vi "Init Interface.vi"(8 "error in":errorcluster, 9 "Config Section":string, 10 "hse-config":refnum<class "config-base.lvclass">, 11 "DB-SQLite":refnum<class "DB-SQLite.lvclass">) -> (0 "error out":errorcluster, 3 "DB-SQLite":refnum<class "DB-SQLite.lvclass">)   [LabVIEW 2020, in "hse-db-sqlite.lvlib" / "DB-SQLite.lvclass"]
doc: "____\nHAMPEL SOFTWARE ENGINEERING v1.4.0 (2023-12-19 09:52)"
uses:
  DB-SQLite.lvclass
  hse-libraries/Source/hse-configuration/config-base/config-base.lvclass
  hse-libraries/Source/hse-application/hse-application.lvclass/hse-application.ctl
  hse-libraries/Source/hse-application/HSE Application not initialized--error.vi
  hse-libraries/Source/hse-application/hse-application__GetSingleton.vi
  <vilib>/Utility/sysdir.llb/Get System Directory.vi
  <vilib>/Utility/error.llb/Error Cluster From Error Code.vi
  DB-SQLite.lvclass/DB-SQLite.ctl
  hse-libraries/Source/hse-application/hse-application.lvclass
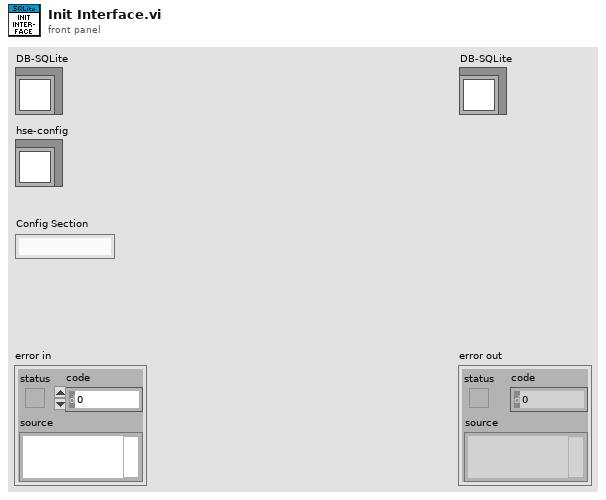
[diagram p1: front panel]
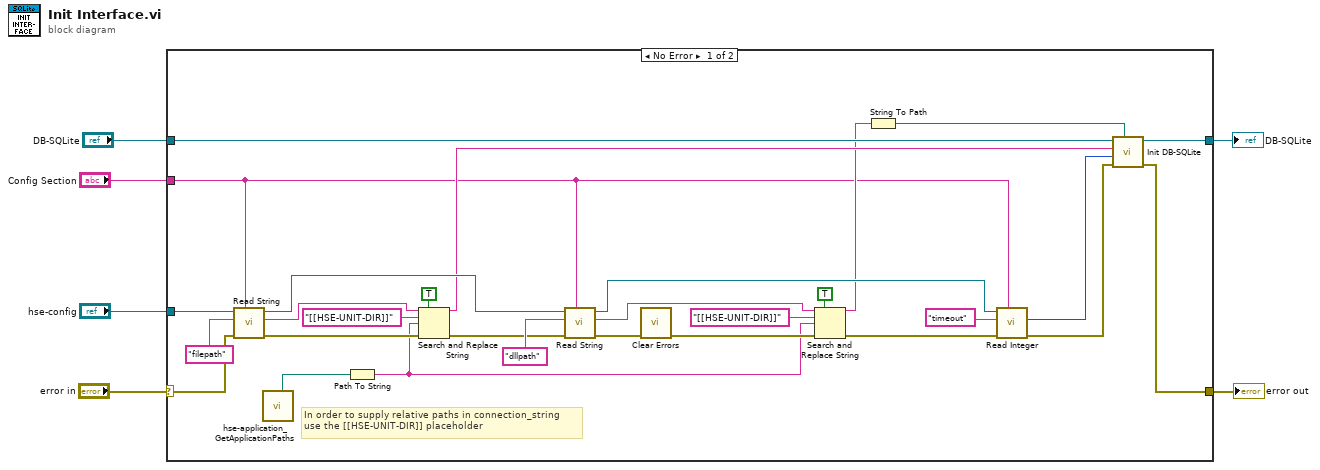
[diagram p0: block diagram]
diagram:
  n1 = case shown="No Error" "error in" {
    selector: "error in" -> [w35 w37]
    tunnel: [w28 w37] -> w5
    tunnel: [w27 w36] -> w1
    tunnel: "DB-SQLite" -> [w30 w36]
    tunnel: "hse-config" -> [w33 _]
    tunnel: "Config Section" -> [w7 _]
    frame No Error {
      # "In order to supply relative paths in connection_string\nuse the [[HSE-UNIT-DIR]] placeholder"
      n2 = call-dynamic "Read String.vi"("Section"=w7, "error in"=w35, "Key"="filepath", "config-base in"=w33) -> ("error out"=w19:errorcluster, "Value"=w18:string, "config-base out"=w23:refnum<class "config-base.lvclass">)  [unwired: 5 in]
      n3 = call "hse-application_GetApplicationPaths.vi"() -> ("Config/Unit Directory"=w20:path)  [unwired: 5 in, 6 out]
      n4 = Path To String(path=w20) -> (string=w12:string)
      n5 = Search and Replace String(replace all?=TRUE ("replace all? (F)"), input string=w18, search string="[[HSE-UNIT-DIR]]" ("Key"), replace string=w12, error in=w19) -> (result string=w17:string, error out=w8:errorcluster)  [unwired: 3 in, 2 out]
      n6 = call-dynamic "Read String.vi"("Section"=w7, "error in"=w8, "Key"="dllpath", "config-base in"=w23) -> ("error out"=w25:errorcluster, "Value"=w10:string, "config-base out"=w24:refnum<class "config-base.lvclass">)  [unwired: 5 in]
      n7 = call <vilib>:"Clear Errors.vi"("error in (no error)"=w25) -> ("error out"=w14:errorcluster)  [unwired: 5 in, 1 out]
      n8 = Search and Replace String(replace all?=TRUE ("replace all? (F)"), input string=w10, search string="[[HSE-UNIT-DIR]]" ("Key"), replace string=w12, error in=w14) -> (result string=w11:string, error out=w13:errorcluster)  [unwired: 3 in, 2 out]
      n9 = String To Path(string=w11) -> (path=w9:path)
      n10 = call-dynamic "Read Integer.vi"("Section"=w7, "error in"=w13, "Key"="timeout", "config-base in"=w24) -> ("error out"=w31:errorcluster, "Value"=w29:i64)  [unwired: 5 in, 1 out]
      n11 = call-dynamic "Init DB-SQLite.vi"("DLL-Filepath"=w9, "error in"=w31, "busy timeout (ms)"=w29, "DB-Filepath"=w17, "DB-SQLite in"=w30) -> ("error out"=w28:errorcluster, "DB-SQLite out"=w27:refnum<class "DB-SQLite.lvclass">)  [unwired: 5 in]
    }
    frame Error {
    }
  }
  "error out" <- w5
  "DB-SQLite" <- w1
